vi "id.Set id type as none.vi"(8 "error in (no error)":errorcluster, 11 "id in":refnum<class "id.lvclass">) -> (0 "error out":errorcluster, 3 "id out":refnum<class "id.lvclass">)   [LabVIEW 2020, in "JSON-RPC Lib.lvlib" / "id.lvclass"]
uses:
  id.lvclass
  id.lvclass/id.ctl
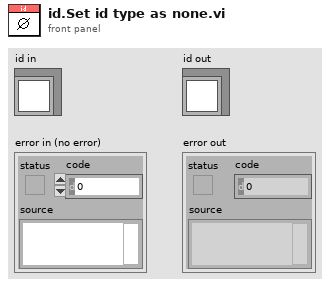
[diagram p1: front panel]
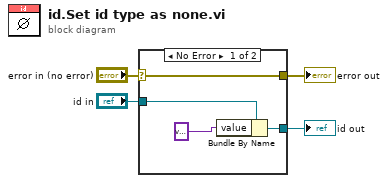
[diagram p0: block diagram]
diagram:
  n1 = case shown="No Error" "error in (no error)" {
    selector: "error in (no error)" -> [w6 w10]
    tunnel: [w6 w10] -> w3
    tunnel: [w7 w9] -> w1
    tunnel: "id in" -> [w8 w9]
    frame No Error {
      n2 = Bundle By Name(cluster=w8, "value"=variant ("JSON Value in")) -> (w7:refnum<class "id.lvclass">)
    }
    frame Error {
    }
  }
  "error out" <- w3
  "id out" <- w1
